vi "ReadSensorValues_v1.2.vi"(1 "VISA resource name":refnum<visa-resource-name>, 2 "sensor type nr":u16, 3 "Sensor Nr":i32) -> ()   [LabVIEW 2012]
uses:
  <vilib>/nican/nicantsk.llb/CAN Interface.ctl
  TimeValue.ctl
  SensorTypes.ctl
  SensorStates.ctl
  <vilib>/nican/nicantsk.llb/CAN Mode.ctl
  <vilib>/nican/nicantsk.llb/CAN Task Reference.ctl
  globalVariables.vi
  <vilib>/Utility/file.llb/Write To Spreadsheet File (string).vi
  <vilib>/nican/nicantsk.llb/CAN Read Multi Chan Single Samp 1D Dbl.vi
  <instrlib>/Agilent 34970/Agilent 34970.lvlib
panel:
  in  "Sensor type":T1
  out "AllValuesOfSensor":T2[](array[typedef])
  in  "Cancel Measurement":bool
  out "new data":bool
  out "Sample number":i32
  in  "CAN Interface":T3 items=["CAN0"=0, "CAN1"=1, "CAN2"=2, "CAN3"=3, "CAN4"=4, "CAN5"=5, "CAN6"=6, "CAN7"=7, "CAN8"=8, "CAN9"=9, "CAN10"=10, "CAN11"=11, "CAN12"=12, "CAN13"=13, "CAN14"=14, "CAN15"=15, "CAN16"=16, "CAN17"=17, "CAN18"=18, "CAN19"=19, "CAN20"=20, "CAN21"=21, "CAN22"=22, "CAN23"=23, "CAN24"=24, "CAN25"=25, "CAN26"=26, "CAN27"=27, "CAN28"=28, "CAN29"=29, "CAN30"=30, "CAN31"=31, "CAN32"=32, "CAN33"=33, "CAN34"=34, "CAN35"=35, "CAN36"=36, "CAN37"=37, "CAN38"=38, "CAN39"=39, "CAN40"=40, "CAN41"=41, "CAN42"=42, "CAN43"=43, "CAN44"=44, "CAN45"=45, "CAN46"=46, "CAN47"=47, "CAN48"=48, "CAN49"=49, "CAN50"=50, "CAN51"=51, "CAN52"=52, "CAN53"=53, "CAN54"=54, "CAN55"=55, "CAN56"=56, "CAN57"=57, "CAN58"=58, "CAN59"=59, "CAN60"=60, "CAN61"=61, "CAN62"=62, "CAN63"=63, "MAX default"=64, "CAN256 (Virtual)"=256, "CAN257 (Virtual)"=257]
  out "Error Flag":bool
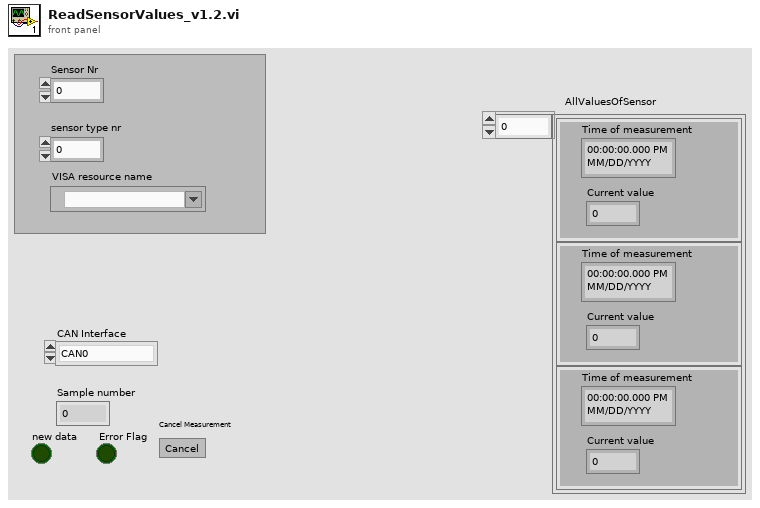
[diagram p1: front panel]
types:
  T1 = typedef "SensorTypes.ctl" = enum16{"IT 600-S (Analogue)", "CAB 300-C SP3 (CAN)", "xyz TODO (PWM)", "xyz TODO (LIN)", "xyz TODO (Analogue)", "difference"}
  T2 = typedef "TimeValue.ctl" = cluster{"Time of measurement":timestamp, "Current value":dbl}
  T3 = typedef "CAN Interface.ctl" = u16
  T4 = typedef "SensorStates.ctl" = enum16{"init", "measure", "terminate"}
  T5 = cluster{"Include Alarm Data F:(No)":bool, "Include Channel # (F:No)":bool, "Include Time (F:No)":bool, "Include Units (F:No)":bool}
  T6 = cluster{"Aperture Value (.4)":dbl, "Aperture (1:Minimum)":u16, "NPLC (1)":u16, "Bandwidth (3 Hz)":u16, "Input Impedance (F:Fixed)":bool, "Integration Time (F:Aperture)":bool}
  T7 = enum16{"100 mV", "1 V", "10 V", "100 V", "300 V", "Minimum", "Maximum"}
  T8 = enum16{"Bus", "Immediate", "External", "Alarm 1", "Alarm 2", "Alarm 3", "Alarm 4", "Timer"}
  T9 = cluster{"Timeout Value (10000)":u32, "Baud Rate (57600)":enum16{"1200", "2400", "4800", "9600", "19200", "38400", "57600", "115200"}, "Flow Control (1:XON/XOFF)":enum16{"None", "XON / XOFF", "RTS / CTS", "DTR / DSR"}}
  T10 = enum16{"Remote Trigger", "Immediate Trigger", "Wait for Trigger", "Abort Scan"}
  T11 = typedef "CAN Task Reference.ctl" = u32
  T12 = typedef "Semaphore RefNum" = refnum<k1>
  T13 = typedef "CAN Mode.ctl" = u16
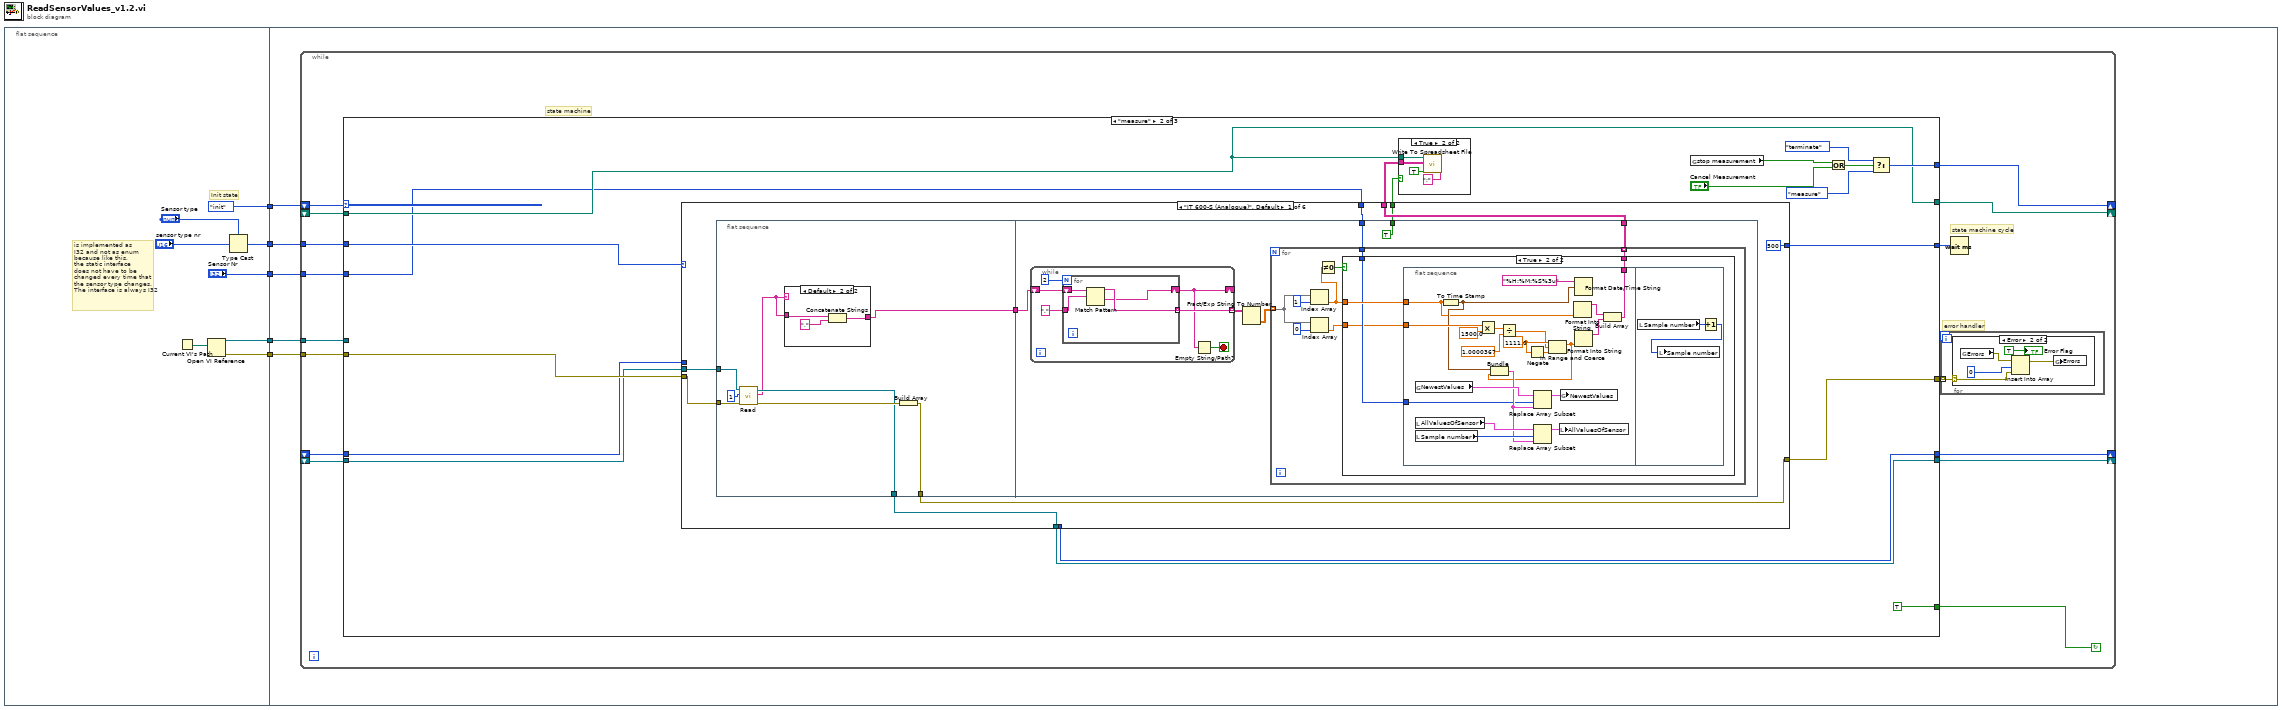
[diagram p0: block diagram]
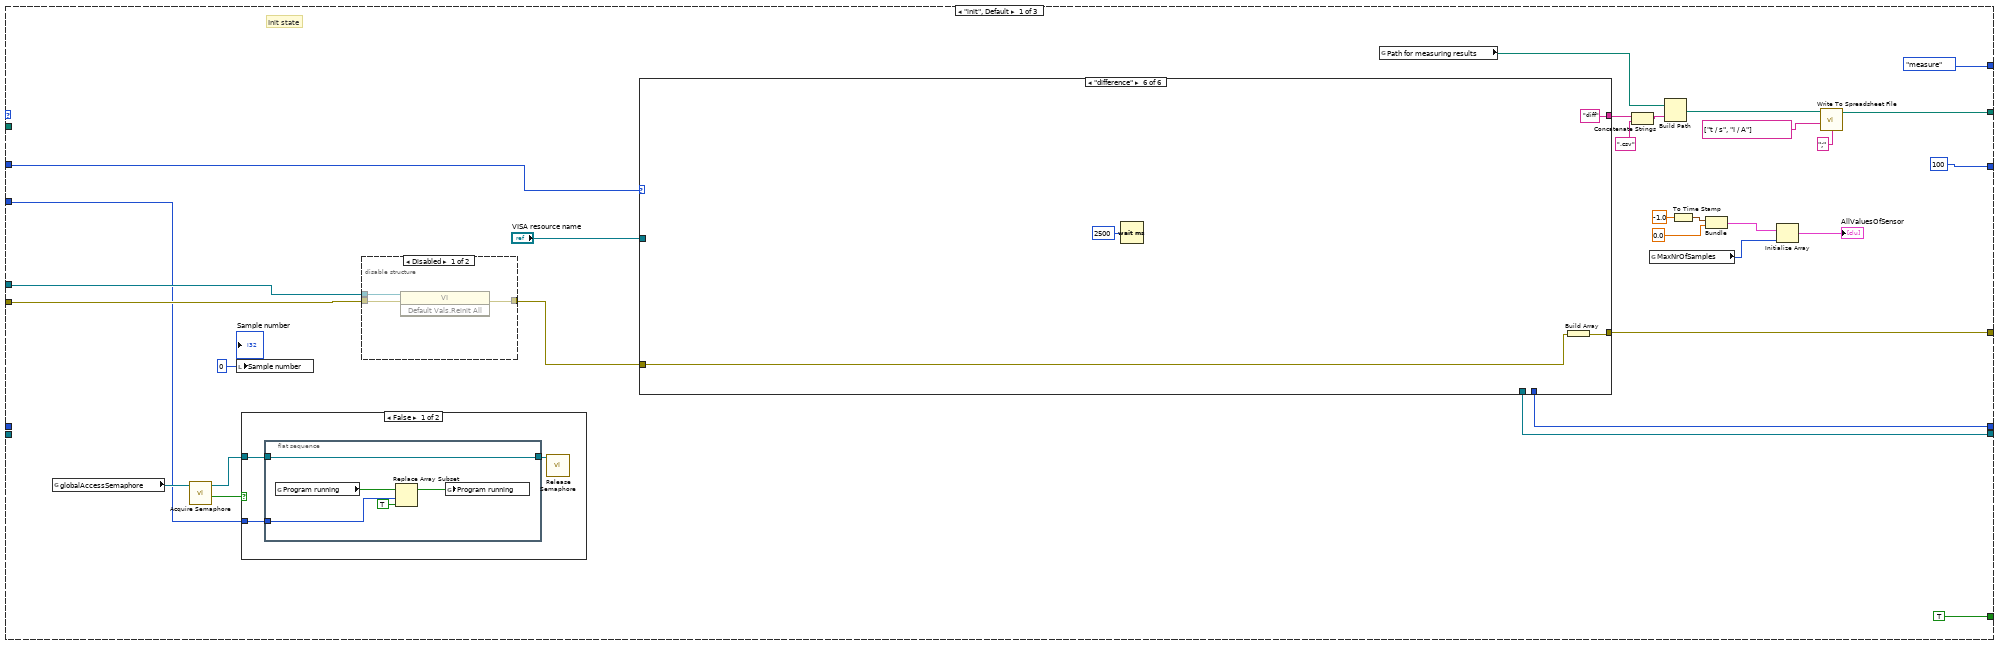
[diagram p3: hidden frame]
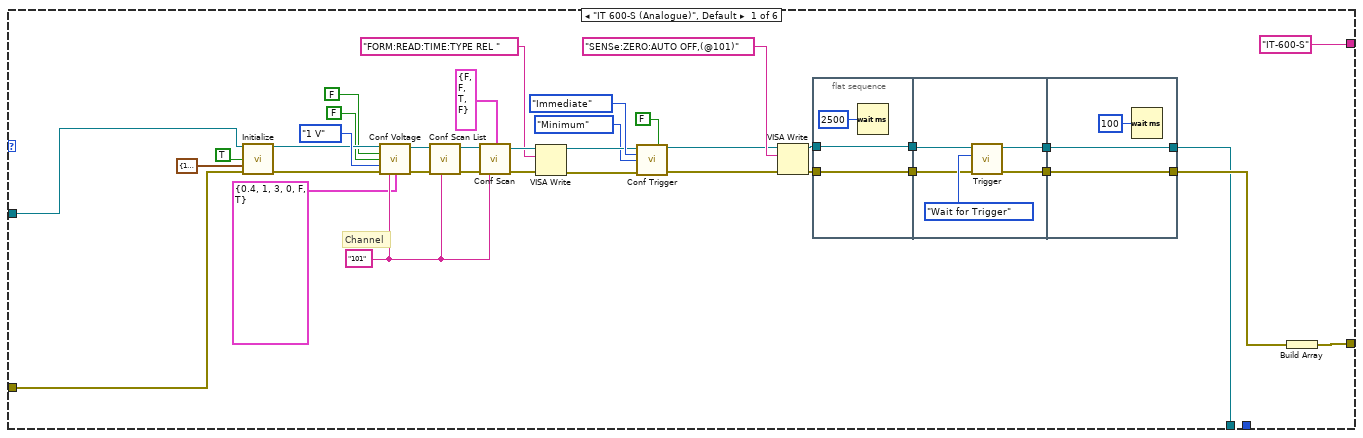
[diagram p6: hidden frame]
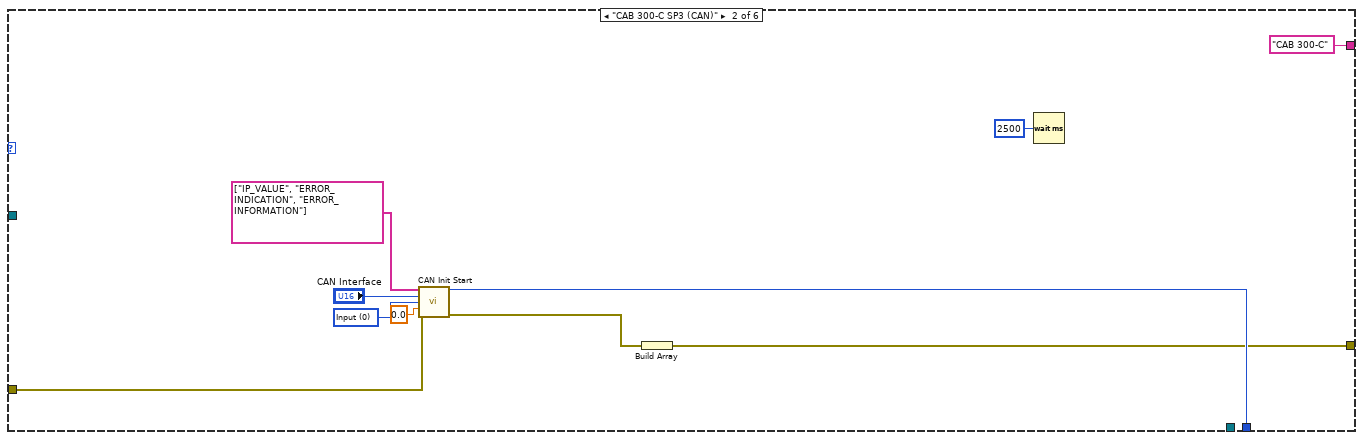
[diagram p7: hidden frame]
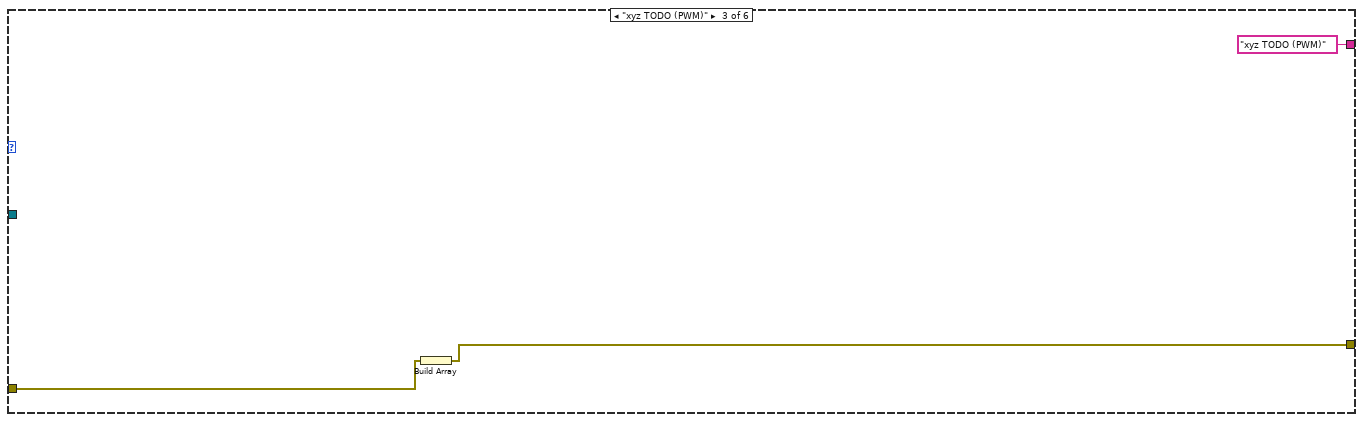
[diagram p8: hidden frame]
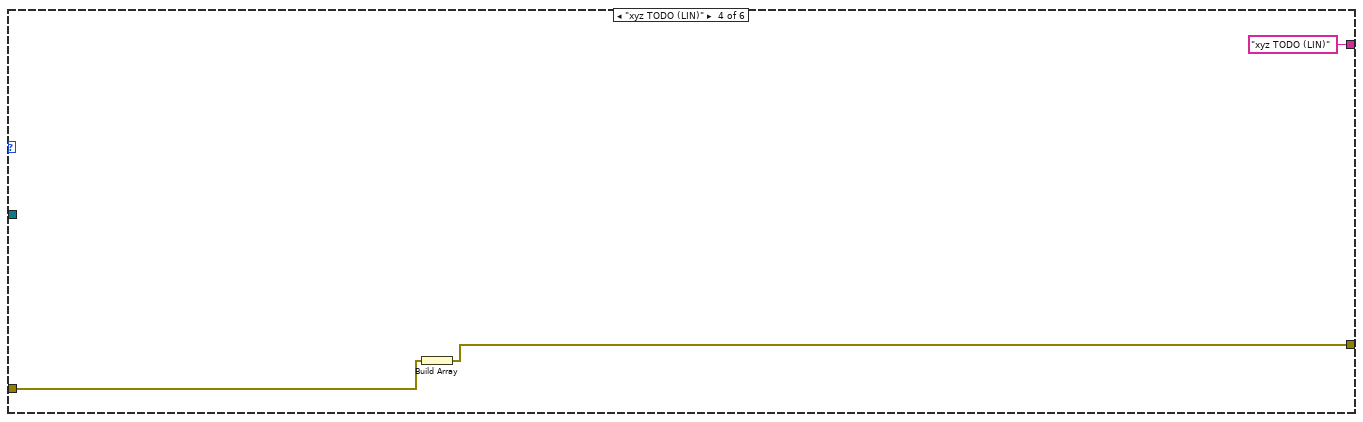
[diagram p9: hidden frame]
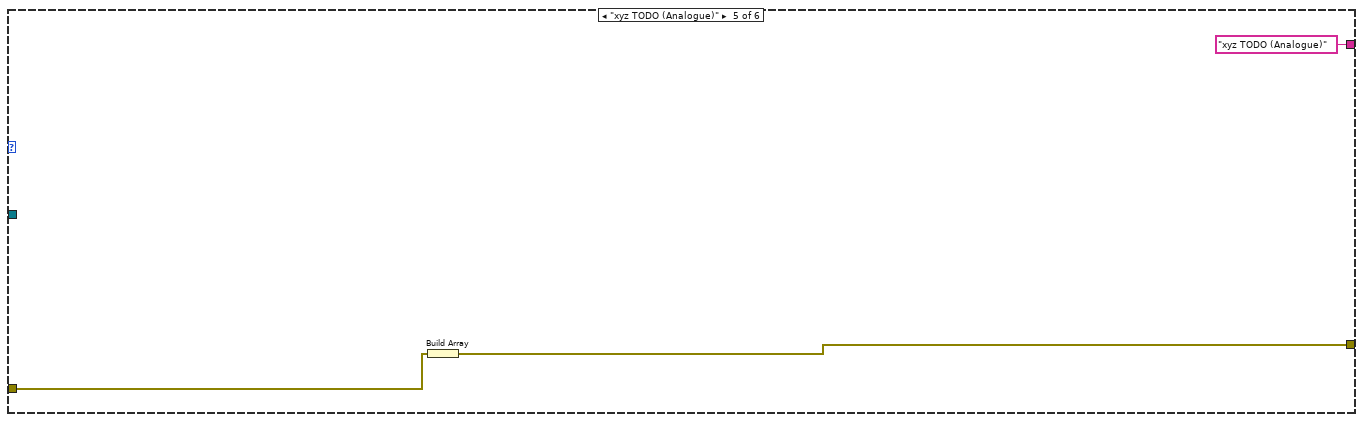
[diagram p10: hidden frame]
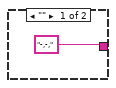
[diagram p12: hidden frame]
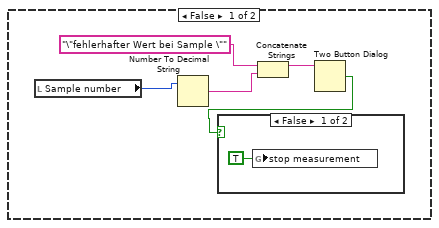
[diagram p13: hidden frame]
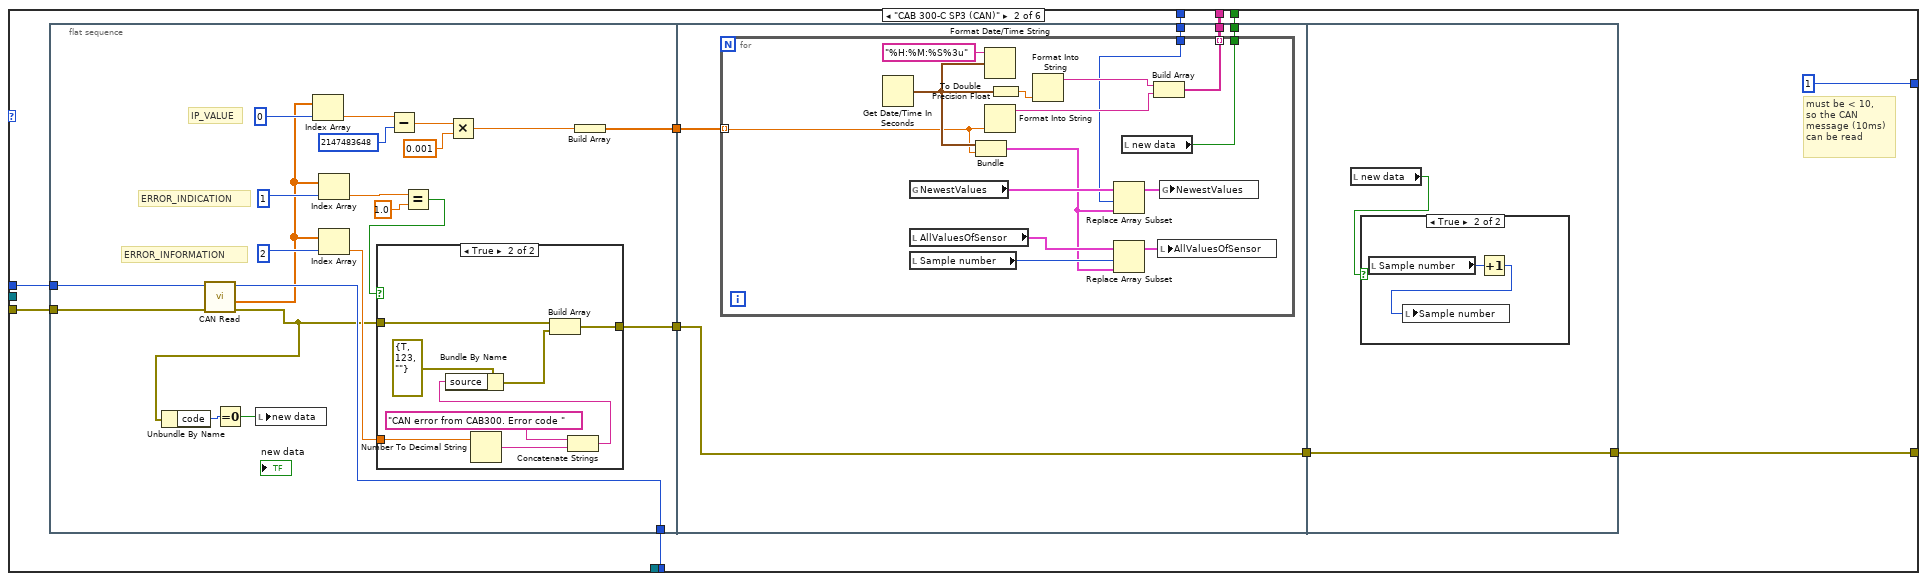
[diagram p15: hidden frame]
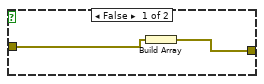
[diagram p16: hidden frame]
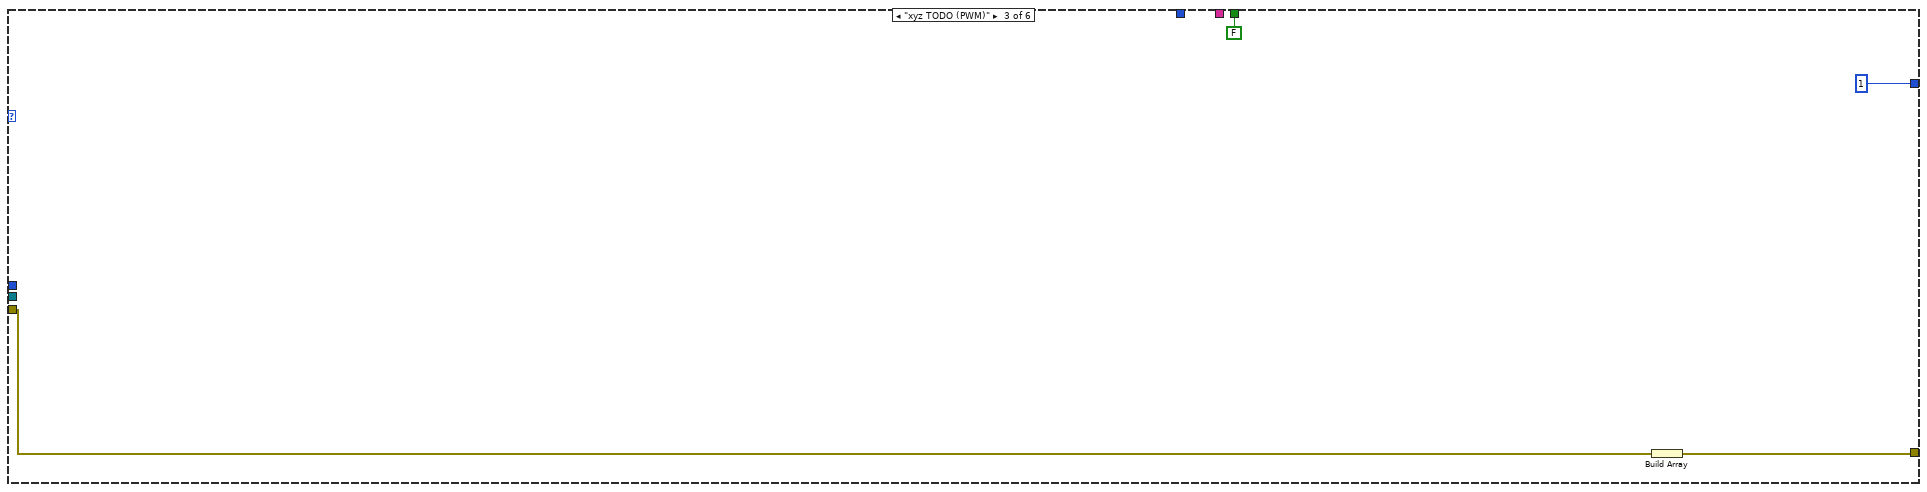
[diagram p18: hidden frame]
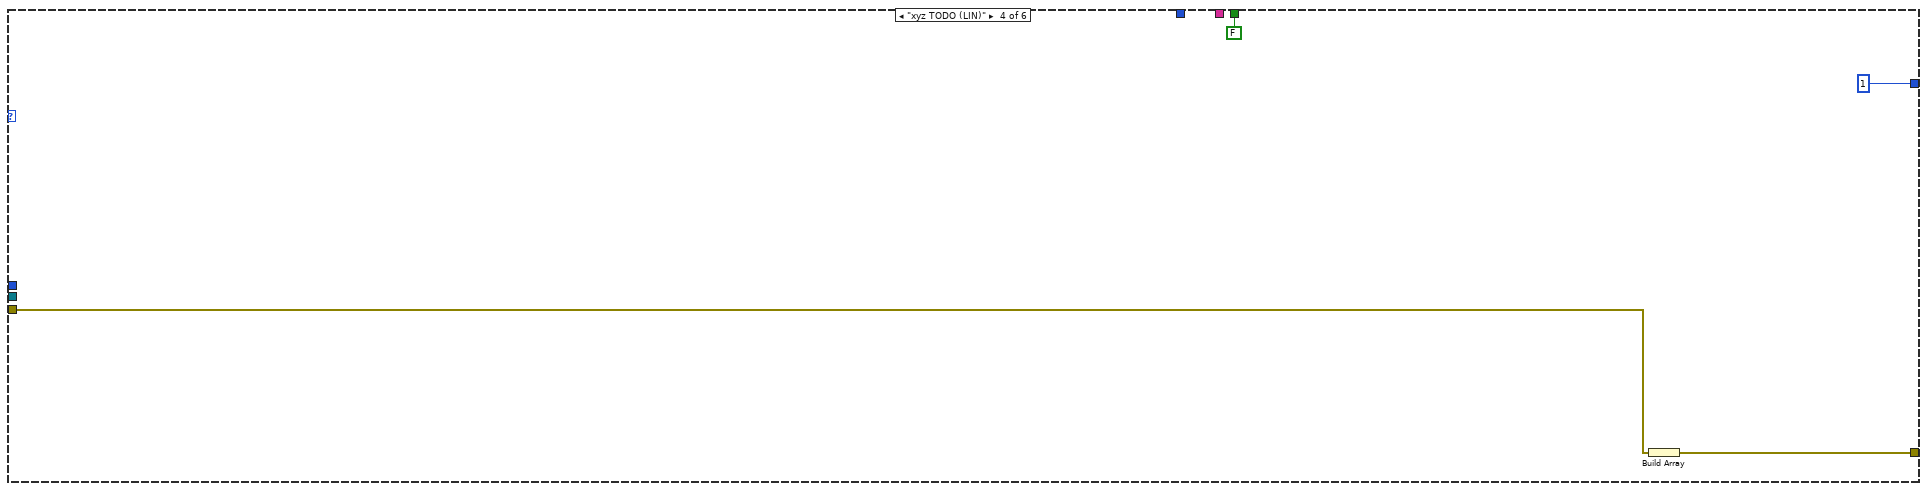
[diagram p19: hidden frame]
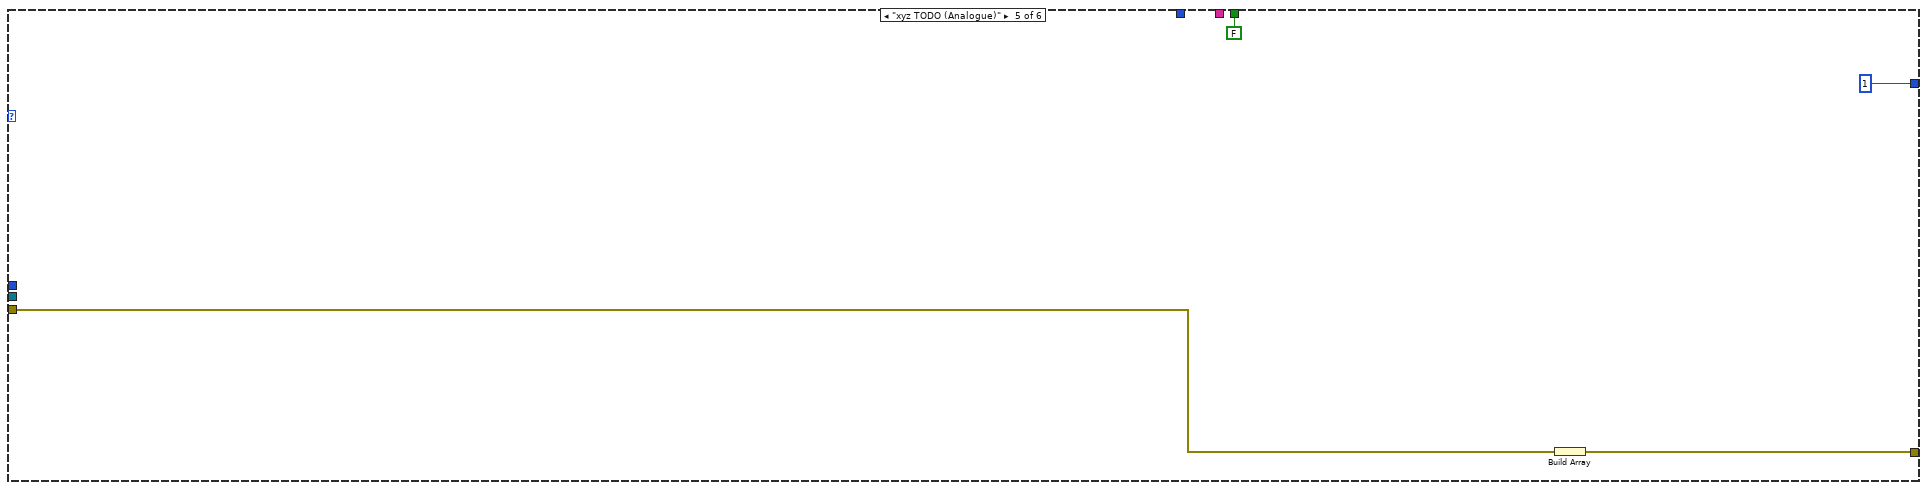
[diagram p20: hidden frame]
diagram:
  n1 = flat-sequence {
    tunnel: [SensorStates."init" ("States IEEE-488")] -> w5
    tunnel: [w13] -> w4
    tunnel: [w12] -> w3
    tunnel: [w6] -> w2
    tunnel: ["Sensor Nr"] -> w1
    tunnel: w5 -> [w16]
    tunnel: w4 -> [w18]
    tunnel: w3 -> [w17]
    tunnel: w2 -> [w15]
    tunnel: w1 -> [w14]
    frame #0 {
      # "is implemented as\nI32 and not as enum \nbecause like this, \nthe static interface \ndoes not have to be \nchanged every time that\nthe sensor type changes.\nThe interface is always I32"
      # "Init state"
      n2 = Current VI's Path() -> (path=w11:path)
      n3 = Open VI Reference(vi path=w11) -> (vi reference=w13:refnum<vi>, error out=w12:errorcluster)  [unwired: 2 in, 3 out]
      n4 = Type Cast(type="Sensor type", x="sensor type nr") -> (*(type *) &x=w6:T1)
    }
    frame #1 {
      n5 = while {
        tunnel: w18 -> [w32]
        tunnel: w17 -> [w31]
        shift-right: [w29] -> _
        shift-left: w16 -> [w30]
        shift-right: [w28] -> _
        shift-left: _ -> [w27]
        tunnel: w15 -> [w25]
        shift-right: [w24] -> _
        shift-left: _ -> [w23]
        shift-right: [w21] -> _
        shift-left: _ -> [w20]
        tunnel: w14 -> [w19]
        stop <- w22 continue-if-true
        # "state machine"
        # "error handler"
        # "state machine cycle"
        n6 = case shown="\"measure\"" w30 {
          tunnel: [u32 100 ("milliseconds to wait") w157 u32 50 ("milliseconds to wait")] -> w33
          tunnel: w32 -> [w67 _ w372]
          tunnel: w31 -> [w68 w167 w376]
          tunnel: [SensorStates."measure" ("States IEEE-488") w168 SensorStates."terminate" ("States IEEE-488")] -> w29
          tunnel: [w65 w163 T11 0 ("task reference out")] -> w28
          tunnel: w27 -> [_ w164 w375]
          tunnel: [w63 w165 w374] -> w26
          tunnel: w25 -> [w41 w153 w360]
          tunnel: [TRUE TRUE FALSE] -> w22
          tunnel: [w59 w158 refnum<visa-resource-name> refnum ("VISA Resource Name Out")] -> w24
          tunnel: w23 -> [_ w159 w369]
          tunnel: [w54 w156 w364] -> w21
          tunnel: w20 -> [_ w156 w364]
          tunnel: w19 -> [w40 w152 w359]
          frame "init", Default {
            # "Init state"
            n7 = global read "globalVariables.vi" "globalAccessSemaphore"() -> (w44:T12)
            n8 = call <vilib>:"Acquire Semaphore.vi"("semaphore"=w44) -> ("timed out"=w42:bool, "semaphore out"=w43:T12)  [unwired: 4 in, 1 out]
            n9 = local write "Sample number"(0 ("Sample number")) -> ()
            n10 = case shown="False" w42 {
              tunnel: w43 -> [w71 _]
              tunnel: w40 -> [w70 _]
              frame False {
                n11 = flat-sequence {
                  tunnel: w71 -> [w77]
                  tunnel: [w77] -> w72
                  tunnel: w70 -> [w73]
                  frame #0 {
                    n12 = global read "globalVariables.vi" "Program running"() -> (w74:bool[])
                    n13 = Replace Array Subset(array=w74, new element=TRUE ("new element/subarray"), index=w73) -> (w75:bool[])
                    n14 = global write "globalVariables.vi" "Program running"(w75) -> ()
                  }
                }
                n15 = call <vilib>:"Release Semaphore.vi"("semaphore"=w72) -> ()  [unwired: 5 in, 2 out]
              }
              frame True {
              }
            }
            n16 = disable-structure shown="Disabled" {
              disable-tunnel: w68 -> [w80 _]
              disable-tunnel: w67 -> [w79 _]
              disable-tunnel: [w78 _] -> w64
              frame Disabled {
                n17 = invoke class="VI" method="Default Vals.Reinit All"(reference=w79, error in=w80) -> (error out=w78:errorcluster)  [unwired: 1 in, 2 out]
              }
              frame Enabled {
              }
            }
            n18 = case shown="\"difference\"" w41 {
              tunnel: [_ w134 _ _ _ _] -> w65
              tunnel: w64 -> [w90 w133 w140 w143 w147 w149]
              tunnel: [w117 w131 w141 w144 w146 w150] -> w63
              tunnel: "VISA resource name" -> [w84 _ _ _ _ _]
              tunnel: [w88 _ _ _ _ _] -> w59
              tunnel: ["IT-600-S" ("name or relative path") "CAB 300-C" ("name or relative path") "xyz TODO (PWM)" ("name or relative path") "xyz TODO (LIN)" ("name or relative path") "xyz TODO (Analogue)" ("name or relative path") "diff" ("name or relative path")] -> w53
              frame "IT 600-S (Analogue)", Default {
                w94 = "101" ("Channel List (Volt.)")
                # "Channel"
                n19 = call <instrlib>:"Initialize.vi"("VISA Resource Name"=w84, "Reset (T: Reset)"=TRUE, "Serial Port Configuration"=T9 {"Timeout Value (10000)"=10000, "Baud Rate (57600)"=enum."57600", "Flow Control (1:XON/XOFF)"=enum."XON / XOFF"}, "error in (no error)"=w90) -> ("VISA Resource Name Out"=w112:refnum<visa-resource-name>, "error out"=w109:errorcluster)  [unwired: 10 in]
                n20 = call <instrlib>:"Conf Voltage.vi"("VISA Resource Name"=w112, "AC/DC (F:DC)"=FALSE, "Autorange? (F:Off)"=FALSE, "Range (6:Max)"=T7."1 V" ("Range (Volt.)"), "error in (no error)"=w109, "Channel List (empty)"=w94, "Advanced Config"=T6 {"Aperture Value (.4)"=0.4, "Aperture (1:Minimum)"=1, "NPLC (1)"=3, "Bandwidth (3 Hz)"=0, "Input Impedance (F:Fixed)"=FALSE, "Integration Time (F:Aperture)"=TRUE}) -> ("VISA Resource Name Out"=w111:refnum<visa-resource-name>, "error out"=w106:errorcluster)  [unwired: 6 in, 1 out]
                n21 = call <instrlib>:"Conf Scan List.vi"("Scan List (empty)"=w94, "error in (no error)"=w106, "VISA Resource Name"=w111) -> ("error out"=w105:errorcluster, "VISA Resource Name Out"=w107:refnum<visa-resource-name>)  [unwired: 6 in, 1 out]
                n22 = call <instrlib>:"Conf Scan.vi"("VISA Resource Name"=w107, "error in (no error)"=w105, "Channel List (empty)"=w94, "Scan Fields"=T5 {"Include Alarm Data F:(No)"=FALSE, "Include Channel # (F:No)"=FALSE, "Include Time (F:No)"=TRUE, "Include Units (F:No)"=FALSE}) -> ("VISA Resource Name Out"=w102:refnum<visa-resource-name>, "error out"=w101:errorcluster)  [unwired: 9 in, 1 out]
                n23 = VISA Write(VISA resource name=w102, write buffer="FORM:READ:TIME:TYPE REL ", error in (no error)=w101) -> (VISA resource name out=w99:refnum<visa-resource-name>, error out=w100:errorcluster)  [unwired: 1 out]
                n24 = call <instrlib>:"Conf Trigger.vi"("VISA Resource Name"=w99, "Wait for Trigger? (F:No)"=FALSE, "Source (1:Immediate)"=T8."Immediate", "Time-Scan Interval (1:Min)"=enum16{"Manual", "Minimum", "Maximum"}."Minimum", "error in (no error)"=w100) -> ("VISA Resource Name Out"=w81:refnum<visa-resource-name>, "error out"=w82:errorcluster)  [unwired: 8 in, 1 out]
                n25 = VISA Write(VISA resource name=w81, write buffer="SENSe:ZERO:AUTO OFF,(@101)", error in (no error)=w82) -> (VISA resource name out=w93:refnum<visa-resource-name>, error out=w92:errorcluster)  [unwired: 1 out]
                n26 = flat-sequence {
                  tunnel: [w119] -> w116
                  tunnel: w93 -> [w119]
                  tunnel: [w118] -> w115
                  tunnel: w92 -> [w118]
                  tunnel: w116 -> [w122]
                  tunnel: w115 -> [w121]
                  tunnel: [w125] -> w87
                  tunnel: [w124] -> w86
                  tunnel: [w127] -> w89
                  tunnel: [w128] -> w88
                  tunnel: w87 -> [w128]
                  tunnel: w86 -> [w127]
                  frame #0 {
                    n27 = Wait (ms)(milliseconds to wait=u32 2500) -> ()  [unwired: 1 out]
                  }
                  frame #1 {
                    n28 = call <instrlib>:"Trigger.vi"("error in (no error)"=w121, "Command (0:Rem Trig)"=T10."Wait for Trigger", "VISA Resource Name"=w122) -> ("error out"=w124:errorcluster, "VISA Resource Name Out"=w125:refnum<visa-resource-name>)  [unwired: 7 in]
                  }
                  frame #2 {
                    n29 = Wait (ms)(milliseconds to wait=u32 100) -> ()  [unwired: 1 out]
                  }
                }
                n30 = Build Array(w89) -> (w117:errorcluster[])
              }
              frame "CAB 300-C SP3 (CAN)" {
                w135 = T13 0 items=["Input", "Output", "Timestamped Input", "Output Recent"] ("mode")
                n31 = call <vilib>:"CAN Init Start.vi"("channel list"=string[] ["IP_VALUE", "ERROR_INDICATION", "ERROR_INFORMATION"] ("Channel List"), "interface"="CAN Interface", "mode"=w135, "sample rate"=0.0, "error in (no error)"=w133) -> ("task reference out"=w134:T11, "error out"=w132:errorcluster)  [unwired: 9 in]
                n32 = Build Array(w132) -> (w131:errorcluster[])
                n33 = Wait (ms)(milliseconds to wait=u32 2500) -> ()  [unwired: 1 out]
              }
              frame "xyz TODO (PWM)" {
                n34 = Build Array(w140) -> (w141:errorcluster[])
              }
              frame "xyz TODO (LIN)" {
                n35 = Build Array(w143) -> (w144:errorcluster[])
              }
              frame "xyz TODO (Analogue)" {
                n36 = Build Array(w147) -> (w146:errorcluster[])
              }
              frame "difference" {
                n37 = Wait (ms)(milliseconds to wait=u32 2500) -> ()  [unwired: 1 out]
                n38 = Build Array(w149) -> (w150:errorcluster[])
              }
            }
            n39 = global read "globalVariables.vi" "Path for measuring results"() -> (w55:path)
            n40 = Concatenate Strings(w53, ".csv" ("string")) -> (w51:string)
            n41 = global read "globalVariables.vi" "MaxNrOfSamples"() -> (w46:i32)
            n42 = Build Path(base path=w55, name or relative path=w51) -> (appended path=w56:path)
            n43 = To Time Stamp(1:-1.0 ("number")) -> (0:w49:timestamp)
            n44 = Bundle(w49, 0.0) -> (w47:cluster{timestamp, dbl})  [unwired: 1 in]
            n45 = Initialize Array(w47, w46) -> (→"AllValuesOfSensor":cluster{timestamp, dbl}[])
            n46 = call-poly <vilib>:"Write To Spreadsheet File.vi"("delimiter (\\t)"=";" ("delimiter (\\t)"), "1D data"=string[] ["t / s", "I / A"], "file path (dialog if empty)"=w56) -> ("new file path (Not A Path if cancelled)"=w54:path)  [unwired: 5 in]
          }
          frame "measure" {
            n47 = case shown="\"IT 600-S (Analogue)\", Default" w153 {
              tunnel: w167 -> [w182 w260 w321 w324 w328 w335]
              tunnel: [w179 w259 w322 w325 w329 w336] -> w165
              tunnel: w164 -> [_ w258 _ _ _ _]
              tunnel: [_ w257 _ _ _ _] -> w163
              tunnel: w159 -> [w183 _ _ _ _ _]
              tunnel: [w180 _ _ _ _ _] -> w158
              tunnel: [u32 500 ("milliseconds to wait") u32 1 ("milliseconds to wait") u32 1 ("milliseconds to wait") u32 1 ("milliseconds to wait") u32 1 ("milliseconds to wait") u32 10 ("milliseconds to wait")] -> w157
              tunnel: [w177 w255 _ _ _ w333] -> w155
              tunnel: [w176 w254 FALSE ("new data") FALSE ("new data") FALSE ("new data") TRUE ("new data")] -> w154
              tunnel: w152 -> [w175 w253 _ _ _ w334]
              frame "IT 600-S (Analogue)", Default {
                n48 = flat-sequence {
                  tunnel: w183 -> [w189]
                  tunnel: w182 -> [w188]
                  tunnel: [w187] -> w181
                  tunnel: [w186] -> w180
                  tunnel: [w185] -> w179
                  tunnel: w181 -> [w201]
                  tunnel: [w198] -> w177
                  tunnel: [TRUE] -> w176
                  tunnel: w175 -> [w196]
                  frame #0 {
                    n49 = call <instrlib>:"Read.vi"("error in (no error)"=w188, "# Channels (1)"=1, "VISA Resource Name"=w189) -> ("error out"=w190:errorcluster, "Readings"=w184:string, "VISA Resource Name Out"=w186:refnum<visa-resource-name>)  [unwired: 5 in, 1 out]
                    n50 = case shown="Default" w184 {
                      tunnel: ["-,-," ("string") w195] -> w187
                      tunnel: w184 -> [_ w194]
                      frame "" {
                      }
                      frame Default {
                        n51 = Concatenate Strings(w194, "," ("string")) -> (w195:string)
                      }
                    }
                    n52 = Build Array(w190) -> (w185:errorcluster[])
                  }
                  frame #1 {
                    n53 = while {
                      tunnel: [w206] -> w200 mode=indexing
                      shift-left: w201 -> [w207]
                      shift-right: [w203] -> _
                      stop <- w205 stop-if-true
                      n54 = for {
                        N: 2 -> [_]
                        tunnel: [w209] -> w206 mode=indexing
                        tunnel: "," ("regular expression") -> [w210]
                        shift-right: [w208] -> w203
                        shift-left: w207 -> [w211]
                        n55 = Match Pattern(string=w211, regular expression=w210) -> (before substring=w209:string, after substring=w208:string)  [unwired: 1 in, 2 out]
                      }
                      n56 = Empty String/Path?(string/path=w203) -> (empty?=w205:bool)
                    }
                    n57 = Fract/Exp String To Number(string=w200) -> (number=w199:dbl[][])  [unwired: 3 in, 1 out]
                    n58 = for {
                      tunnel: w199 -> [w217] mode=indexing
                      tunnel: [w214] -> w198 mode=indexing
                      tunnel: w196 -> [w212]
                      n59 = Index Array(array=w217, index=1 ("disabled index (col)")) -> (element=w215:dbl)
                      n60 = Index Array(array=w217, index=0 ("disabled index (col)")) -> (element=w216:dbl)
                      n61 = Not Equal To 0?(x=w215) -> (x != 0?=w213:bool)
                      n62 = case shown="True" w213 {
                        tunnel: w215 -> [_ w229]
                        tunnel: w216 -> [_ w226]
                        tunnel: [_ w228] -> w214
                        tunnel: w212 -> [_ w227]
                        frame False {
                          n63 = local read "Sample number"() -> (w224:i32)
                          n64 = Number To Decimal String(number=w224) -> (decimal integer string=w221:string)  [unwired: 1 in]
                          n65 = Concatenate Strings("\"fehlerhafter Wert bei Sample \"" ("message"), w221) -> (w223:string)
                          n66 = Two Button Dialog(message=w223) -> (T button?=w220:bool)  [unwired: 2 in]
                          n67 = case shown="False" w220 {
                            frame False {
                              n68 = global write "globalVariables.vi" "stop measurement"(TRUE ("stop measurement")) -> ()
                            }
                            frame True {
                            }
                          }
                        }
                        frame True {
                          n69 = flat-sequence {
                            tunnel: w229 -> [w235]
                            tunnel: w226 -> [w247]
                            tunnel: [w244] -> w228
                            tunnel: w227 -> [w234]
                            frame #0 {
                              w232 = 1111.0 ("x")
                              n70 = global read "globalVariables.vi" "NewestValues"() -> (w238:T2[])
                              n71 = local read "AllValuesOfSensor"() -> (w243:T2[])
                              n72 = local read "Sample number"() -> (w242:i32)
                              n73 = To Time Stamp(1:w235) -> (0:w241:timestamp)
                              n74 = Multiply(x=w247, y=1500.0) -> (x*y=w248:dbl)
                              n75 = Divide(x=w248, y=1.0000367) -> (x/y=w230:dbl)
                              n76 = Negate(x=w232) -> (-x=w233:dbl)
                              n77 = In Range and Coerce(upper limit=w232, x=w230, lower limit=w233) -> (coerced(x)=w231:dbl)  [unwired: 1 out]
                              n78 = Bundle(w241, "x"=w231) -> (w237:cluster{timestamp, "x":dbl})  [unwired: 1 in]
                              n79 = Replace Array Subset(array=w238, new element=w237, index=w234) -> (w239:T2[])
                              n80 = Replace Array Subset(array=w243, new element=w237, index=w242) -> (w240:T2[])
                              n81 = local write "AllValuesOfSensor"(w240) -> ()
                              n82 = global write "globalVariables.vi" "NewestValues"(w239) -> ()
                              n83 = Format Into String(w235) -> (resulting string=w236:string)  [unwired: 3 in, 1 out]
                              n84 = Format Date/Time String(time format string (%c)="%H:%M:%S%3u", seconds (now)=w241) -> ()  [unwired: 1 in, 1 out]
                              n85 = Format Into String(w231) -> (resulting string=w245:string)  [unwired: 3 in, 1 out]
                              n86 = Build Array(w236, w245) -> (w244:string[])
                            }
                            frame #1 {
                              n87 = local read "Sample number"() -> (w252:i32)
                              n88 = Increment(x=w252) -> (x+1=w251:i32)
                              n89 = local write "Sample number"(w251) -> ()
                            }
                          }
                        }
                      }
                    }
                  }
                }
              }
              frame "CAB 300-C SP3 (CAN)" {
                # "must be < 10,\nso the CAN \nmessage (10ms) \ncan be read"
                n90 = flat-sequence {
                  tunnel: [w283] -> w263
                  tunnel: [w282] -> w262
                  tunnel: w260 -> [w284]
                  tunnel: w258 -> [w281]
                  tunnel: [w280] -> w257
                  tunnel: w263 -> [w299]
                  tunnel: w262 -> [w298]
                  tunnel: [w299] -> w261
                  tunnel: [w297] -> w255
                  tunnel: [w296] -> w254
                  tunnel: w253 -> [w295]
                  tunnel: w261 -> [w316]
                  tunnel: [w316] -> w259
                  frame #0 {
                    # "ERROR_INFORMATION"
                    # "ERROR_INDICATION"
                    # "IP_VALUE"
                    n91 = call-poly <vilib>:"CAN Read.vi"("error in (no error)"=w284, "task reference in"=w281) -> ("error out"=w271:errorcluster, "multi-chan single-samp 1D dbl"=w274:dbl[], "task reference out"=w280:T11)  [unwired: 6 in, 1 out]
                    n92 = Unbundle By Name(w271) -> ("code"=w270:i32)
                    n93 = Equal To 0?(x=w270) -> (x = 0?=w269:bool)
                    n94 = local write "new data"(w269) -> ()
                    n95 = Index Array(array=w274, index=0) -> (element=w268:dbl)
                    n96 = Index Array(array=w274, index=1) -> (element=w276:dbl)
                    n97 = Index Array(array=w274, index=2) -> (element=w273:dbl)
                    n98 = Subtract(x=w268, y=u32 2147483648) -> (x-y=w266:dbl)
                    n99 = Equal?(x=w276, y=1.0) -> (x = y?=w272:bool)
                    n100 = case shown="True" w272 {
                      tunnel: w271 -> [w286 w294]
                      tunnel: [w285 w293] -> w283
                      tunnel: w273 -> [_ w288]
                      frame False {
                        n101 = Build Array(w286) -> (w285:errorcluster[])
                      }
                      frame True {
                        n102 = Number To Decimal String(number=w288) -> (decimal integer string=w289:string)  [unwired: 1 in]
                        n103 = Concatenate Strings("CAN error from CAB300. Error code ", w289) -> (w287:string)
                        n104 = Bundle By Name(cluster=errorcluster {"status"=TRUE, "code"=123, "source"=""} ("error out"), "source"=w287) -> (w291:errorcluster)
                        n105 = Build Array(w294, w291) -> (w293:errorcluster[])
                      }
                    }
                    n106 = Multiply(x=w266, y=0.001) -> (x*y=w264:dbl)
                    n107 = Build Array(w264) -> (w282:dbl[])
                  }
                  frame #1 {
                    n108 = for {
                      tunnel: w298 -> [w300] mode=indexing
                      tunnel: [w312] -> w297 mode=indexing
                      tunnel: [w305] -> w296
                      tunnel: w295 -> [w301]
                      n109 = Get Date/Time In Seconds() -> (seconds since 1Jan1904=w303:timestamp)
                      n110 = global read "globalVariables.vi" "NewestValues"() -> (w307:T2[])
                      n111 = local read "AllValuesOfSensor"() -> (w311:T2[])
                      n112 = local read "Sample number"() -> (w310:i32)
                      n113 = Bundle("seconds since 1Jan1904"=w303, w300) -> (w306:cluster{"seconds since 1Jan1904":timestamp, dbl})  [unwired: 1 in]
                      n114 = Format Date/Time String(time format string (%c)="%H:%M:%S%3u", seconds (now)=w303) -> ()  [unwired: 1 in, 1 out]
                      n115 = Format Into String(w300) -> (resulting string=w313:string)  [unwired: 3 in, 1 out]
                      n116 = To Double Precision Float(number=w303) -> (double precision float=w302:dbl)
                      n117 = Format Into String(w302) -> (resulting string=w304:string)  [unwired: 3 in, 1 out]
                      n118 = Replace Array Subset(array=w307, new element=w306, index=w301) -> (w308:T2[])
                      n119 = Replace Array Subset(array=w311, new element=w306, index=w310) -> (w309:T2[])
                      n120 = local read "new data"() -> (w305:bool)
                      n121 = Build Array(w304, w313) -> (w312:string[])
                      n122 = local write "AllValuesOfSensor"(w309) -> ()
                      n123 = global write "globalVariables.vi" "NewestValues"(w308) -> ()
                    }
                  }
                  frame #2 {
                    n124 = local read "new data"() -> (w315:bool)
                    n125 = case shown="True" w315 {
                      frame False {
                      }
                      frame True {
                        n126 = local read "Sample number"() -> (w318:i32)
                        n127 = Increment(x=w318) -> (x+1=w317:i32)
                        n128 = local write "Sample number"(w317) -> ()
                      }
                    }
                  }
                }
              }
              frame "xyz TODO (PWM)" {
                n129 = Build Array(w321) -> (w322:errorcluster[])
              }
              frame "xyz TODO (LIN)" {
                n130 = Build Array(w324) -> (w325:errorcluster[])
              }
              frame "xyz TODO (Analogue)" {
                n131 = Build Array(w328) -> (w329:errorcluster[])
              }
              frame "difference" {
                n132 = flat-sequence {
                  tunnel: w334 -> [w351]
                  tunnel: [w338] -> w333
                  frame #0 {
                    n133 = global read "globalVariables.vi" "NewestValues"() -> (w350:T2[])
                    n134 = local read "AllValuesOfSensor"() -> (w356:T2[])
                    n135 = local read "Sample number"() -> (w355:i32)
                    n136 = Get Date/Time In Seconds() -> (seconds since 1Jan1904=w340:timestamp)
                    n137 = Index Array(array=w350, index #1=1 ("index"), index #2=0 ("index")) -> (element #1=w347:T2, element #2=w346:T2)
                    n138 = To Double Precision Float(number=w340) -> (double precision float=w342:dbl)
                    n139 = Unbundle By Name(w347) -> ("Current value"=w345:dbl)
                    n140 = Unbundle By Name(w346) -> ("Current value"=w344:dbl)
                    n141 = Format Into String(w342) -> (resulting string=w341:string)  [unwired: 3 in, 1 out]
                    n142 = Subtract(x=w345, y=w344) -> (x-y=w339:dbl)
                    n143 = Bundle("seconds since 1Jan1904"=w340, w339) -> (w352:cluster{"seconds since 1Jan1904":timestamp, dbl})  [unwired: 1 in]
                    n144 = Format Into String(w339) -> (resulting string=w343:string)  [unwired: 3 in, 1 out]
                    n145 = Replace Array Subset(array=w350, new element=w352, index=w351) -> (w353:T2[])
                    n146 = Replace Array Subset(array=w356, new element=w352, index=w355) -> (w354:T2[])
                    n147 = local write "AllValuesOfSensor"(w354) -> ()
                    n148 = global write "globalVariables.vi" "NewestValues"(w353) -> ()
                    n149 = Build Array(w341, w343) -> (w337:string[])
                    n150 = Build Array(w337) -> (w338:string[][])
                  }
                  frame #1 {
                    n151 = local read "Sample number"() -> (w358:i32)
                    n152 = Increment(x=w358) -> (x+1=w357:i32)
                    n153 = local write "Sample number"(w357) -> ()
                  }
                }
                n154 = Build Array(w335) -> (w336:errorcluster[])
              }
            }
            n155 = case shown="True" w154 {
              tunnel: w156 -> [_ w172]
              tunnel: w155 -> [_ w171]
              frame False {
              }
              frame True {
                n156 = call-poly <vilib>:"Write To Spreadsheet File.vi"("delimiter (\\t)"=";" ("delimiter (\\t)"), "append to file? (new file:F)"=TRUE, "2D data"=w171, "file path (dialog if empty)"=w172) -> ()  [unwired: 4 in, 1 out]
              }
            }
            n157 = global read "globalVariables.vi" "stop measurement"() -> (w162:bool)
            n158 = Or(x=w162, y="Cancel Measurement") -> (x .or. y?=w160:bool)
            n159 = Select(t=SensorStates."terminate" ("States IEEE-488"), s=w160, f=SensorStates."measure" ("States IEEE-488")) -> (s? t:f=w168:T4)
          }
          frame "terminate" {
            n160 = global read "globalVariables.vi" "Program running"() -> (w367:bool[])
            n161 = Replace Array Subset(array=w367, new element=FALSE ("new element/subarray"), index=w359) -> (w366:bool[])
            n162 = global write "globalVariables.vi" "Program running"(w366) -> ()
            n163 = case shown="\"difference\"" w360 {
              tunnel: w376 -> [w393 w399 w400 w401 w402 w403]
              tunnel: [w392 w398 w400 w401 w402 w403] -> w371
              tunnel: w375 -> [_ w397 _ _ _ _]
              tunnel: w369 -> [w391 _ _ _ _ _]
              frame "IT 600-S (Analogue)", Default {
                n164 = call <instrlib>:"Trigger.vi"("error in (no error)"=w393, "Command (0:Rem Trig)"=T10."Abort Scan", "VISA Resource Name"=w391) -> ("error out"=w395:errorcluster, "VISA Resource Name Out"=w394:refnum<visa-resource-name>)  [unwired: 7 in]
                n165 = call <instrlib>:"Close.vi"("VISA Resource Name"=w394, "error in (no error)"=w395) -> ("error out"=w392:errorcluster)  [unwired: 13 in]
              }
              frame "CAB 300-C SP3 (CAN)" {
                n166 = call <vilib>:"CAN Clear.vi"("error in (no error)"=w399, "task reference in"=w397) -> ("error out"=w398:errorcluster)  [unwired: 9 in]
              }
              frame "xyz TODO (PWM)" {
              }
              frame "xyz TODO (LIN)" {
              }
              frame "xyz TODO (Analogue)" {
              }
              frame "difference" {
              }
            }
            n167 = global read "globalVariables.vi" "globalAccessSemaphore"() -> (w363:T12)
            n168 = call <vilib>:"Acquire Semaphore.vi"("semaphore"=w363) -> ("timed out"=w361:bool, "semaphore out"=w362:T12)  [unwired: 4 in, 1 out]
            n169 = case shown="False" w361 {
              tunnel: w362 -> [w381 _]
              tunnel: w359 -> [w380 _]
              frame False {
                n170 = flat-sequence {
                  tunnel: w381 -> [w390]
                  tunnel: [w390] -> w382
                  tunnel: w380 -> [w383]
                  frame #0 {
                    n171 = local read "AllValuesOfSensor"() -> (w387:T2[])
                    n172 = global read "globalVariables.vi" "AllValues"() -> (w385:T2[][])
                    n173 = Build Array(w387) -> (w388:T2[][])
                    n174 = Transpose 2D Array(2D array=w388) -> (transposed array=w389:T2[][])
                    n175 = Replace Array Subset(array=w385, new element=w389, index (row)=0 ("disabled index (row)"), index (col)=w383) -> (w384:T2[][])
                    n176 = global write "globalVariables.vi" "AllValues"(w384) -> ()
                  }
                }
                n177 = call <vilib>:"Release Semaphore.vi"("semaphore"=w382) -> ()  [unwired: 5 in, 2 out]
              }
              frame True {
              }
            }
            n178 = Close Reference(reference=w372, error in (no error)=w371) -> (error out=w378:errorcluster)
            n179 = Build Array(w378) -> (w374:errorcluster[])
          }
        }
        n180 = for {
          tunnel: w26 -> [w34] mode=indexing
          n181 = case shown="Error" w34 {
            selector: w34 -> [_ w38]
            frame No Error {
            }
            frame Error {
              n182 = global read "globalVariables.vi" "Errors"() -> (w36:errorcluster[])
              n183 = Insert Into Array(array=w36, index=0, new element=w38) -> (w35:errorcluster[])
              n184 = global write "globalVariables.vi" "Errors"(w35) -> ()
              "Error Flag" <- TRUE ("Error Flag")
            }
          }
        }
        n185 = Wait (ms)(milliseconds to wait=w33) -> ()  [unwired: 1 out]
      }
    }
  }
